vi "EXO2-Sonde Serial thread.vi"() -> ()   [LabVIEW 2016, in "EXO2-Sonde.lvlib"]
uses:
  EXO2-Sonde.lvlib
  <vilib>/Utility/miscctls.llb/LVPointTypeDef.ctl
  Var/Holding Var.vi
  <vilib>/Instr/_visa.llb/VISA Configure Serial Port (Instr).vi
  Var/Input Var.vi
panel:
  in  "停止按钮":bool
  in  "启动按钮":bool
  in  "baud rate (9600)":u32=38400
  out "EXO message":T1
  out "EXO原始数据包":string
  out "收到监测数据":bool
  in  "EXO串口":refnum<visa-resource-name>="COM4"
  in  "EXO启用":bool
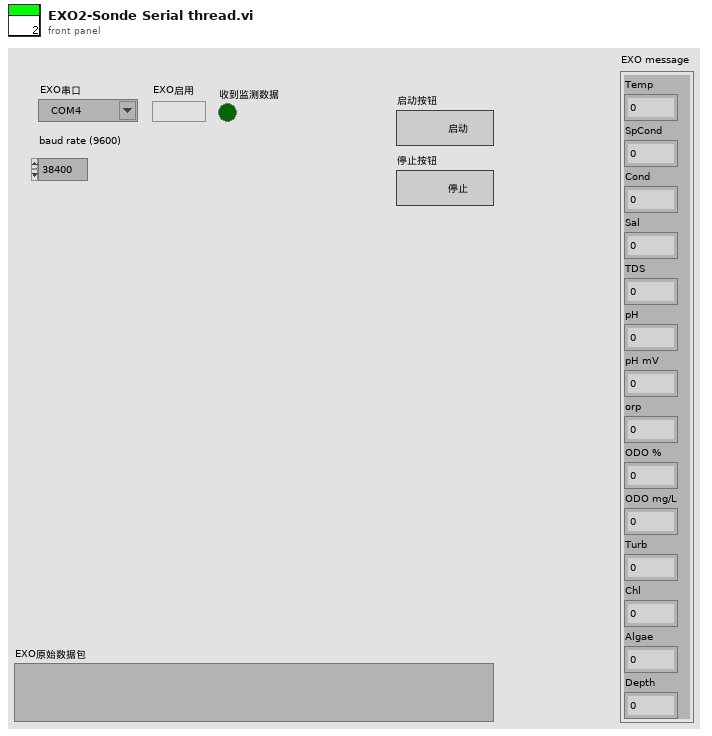
[diagram p1: front panel]
types:
  T1 = cluster{"Temp":dbl, "SpCond":dbl, "Cond":dbl, "Sal":dbl, "TDS":dbl, "pH":dbl, "pH mV":dbl, "orp":dbl, "ODO %":dbl, "ODO mg/L":dbl, "Turb":dbl, "Chl":dbl, "Algae":dbl, "Depth":dbl}
  T2 = enum8{"Enabled", "Disabled", "Disabled and Grayed Out"}
  T3 = typedef "LVPointTypeDef.ctl" = cluster{"Horizontal":i16, "Vertical":i16}
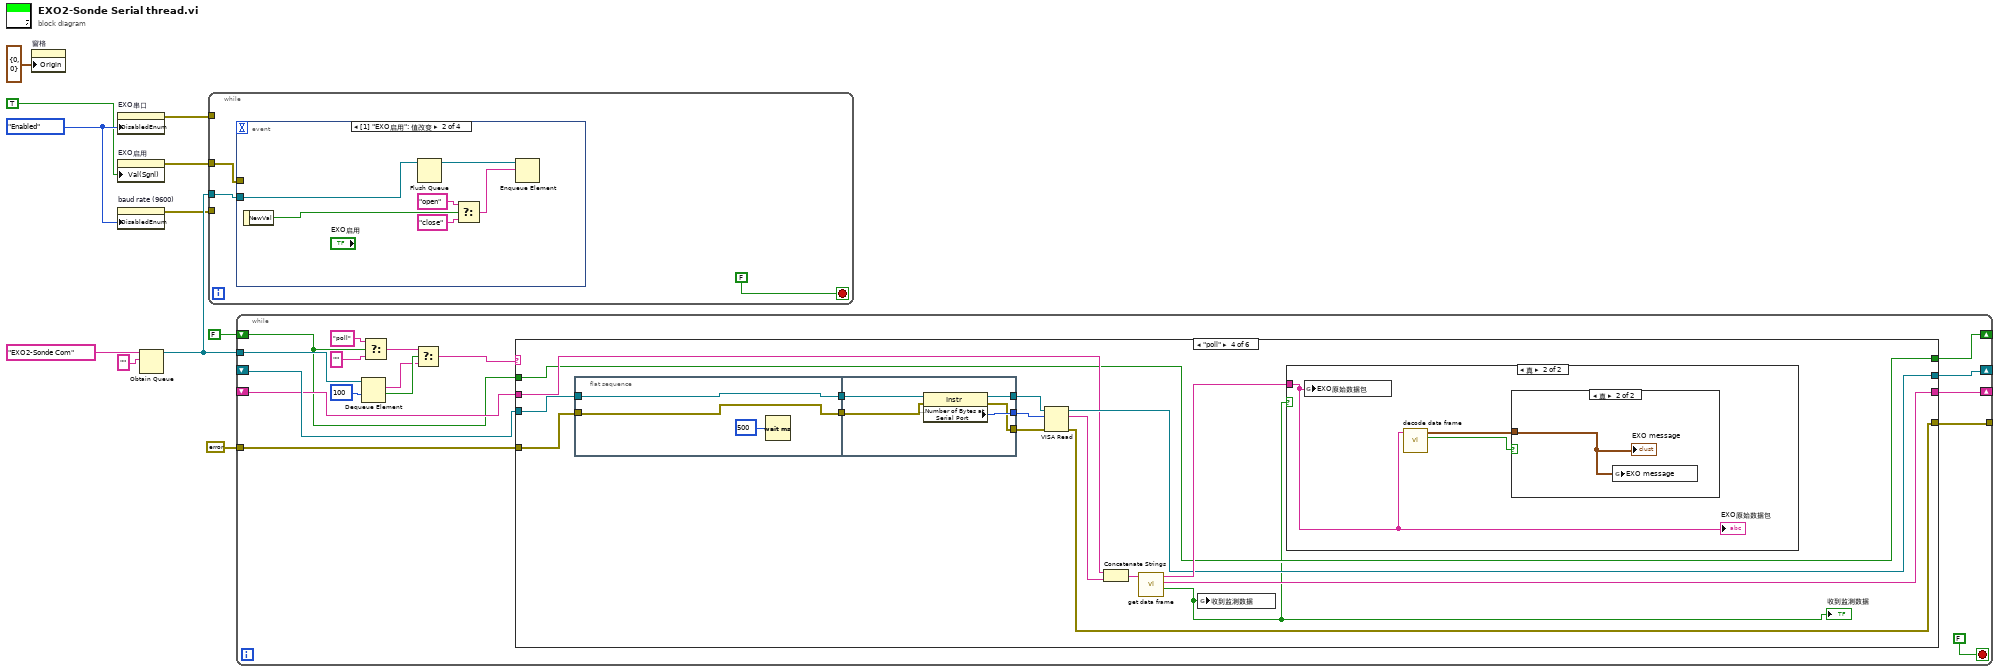
[diagram p0: block diagram]
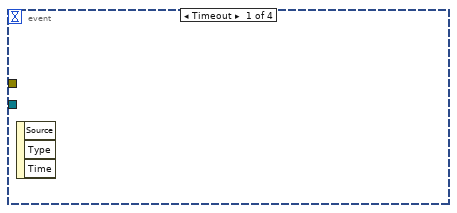
[diagram p2: hidden frame]
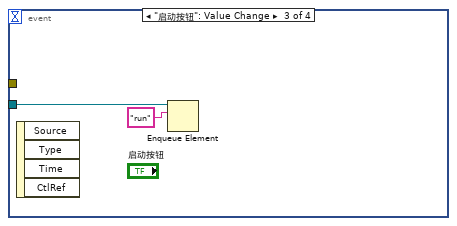
[diagram p3: hidden frame]
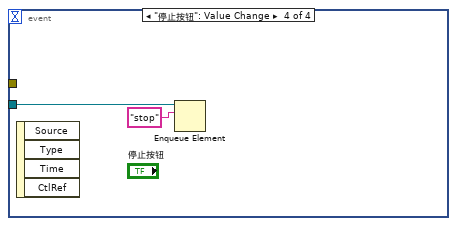
[diagram p4: hidden frame]
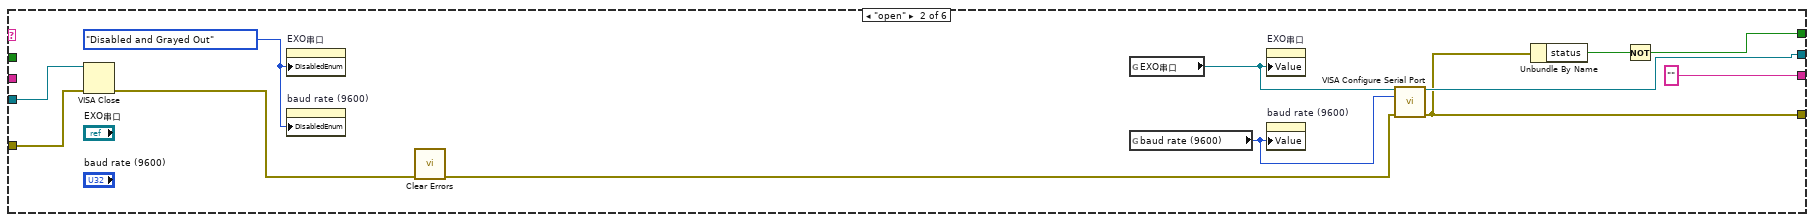
[diagram p6: hidden frame]
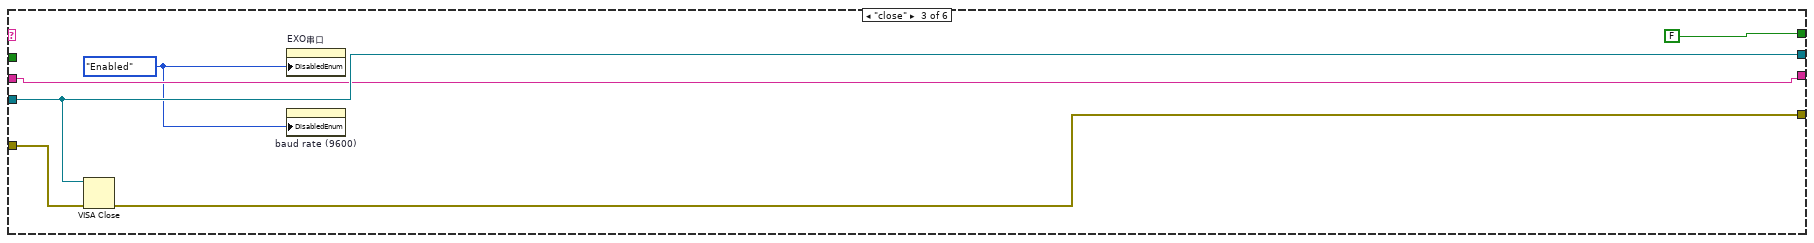
[diagram p7: hidden frame]
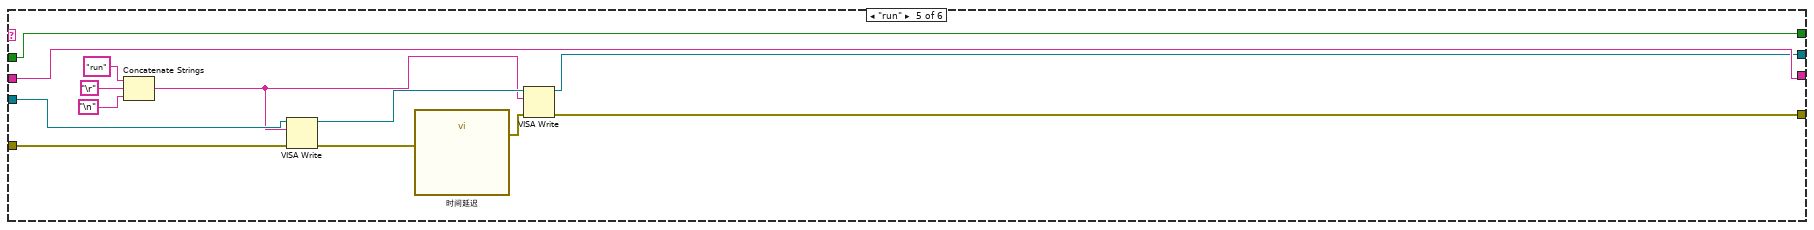
[diagram p10: hidden frame]
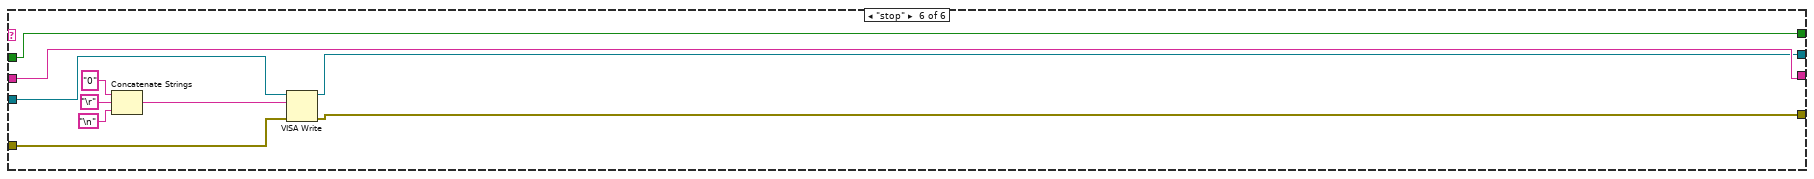
[diagram p11: hidden frame]
diagram:
  w5 = T2."Enabled" ("禁用")
  n1 = property on="窗格" class="Pane"("Origin"=T3 {"Horizontal"=0, "Vertical"=0} ("原点")) -> ()  [unwired: 2 in, 2 out]
  n2 = property on="EXO串口" class="VISAName"("DisabledEnum"=w5) -> (error out=w6:errorcluster)  [unwired: 2 in, 1 out]
  n3 = property on="EXO启用" class="Bool (严格)"("Val(Sgnl)"=TRUE ("值(信号)")) -> (error out=w2:errorcluster)  [unwired: 2 in, 1 out]
  n4 = property on="baud rate (9600)" class="DigNum (严格)"("DisabledEnum"=w5) -> (error out=w4:errorcluster)  [unwired: 2 in, 1 out]
  n5 = Obtain Queue(name (unnamed)="EXO2-Sonde Com" ("名称（未命名）"), element data type="") -> (queue out=w8:refnum<queue>)  [unwired: 3 in, 2 out]
  n6 = while {
    tunnel: w8 -> [w13]
    tunnel: w6 -> [_]
    tunnel: w4 -> [_]
    tunnel: w2 -> [w12]
    stop <- FALSE stop-if-true
    n7 = event shown="[1] \"EXO启用\": 值改变" {
      selector: _ -> [_ _ _ _]
      dyn-events: _ -> [_ _ _ _]
      timeout: _ -> [_ _ _ _]
      tunnel: w13 -> [_ w20 w22 w24]
      tunnel: w12 -> [_ _ _ _]
      event Timeout {
        n8 = event-data() -> ()  [unwired: 1 in, 3 out]
      }
      event "EXO启用": Value Change {
        n9 = event-data() -> ("NewVal"=w19:bool)  [unwired: 1 in]
        n10 = Flush Queue(queue=w20) -> (queue out=w16:refnum<queue>)  [unwired: 1 in, 2 out]
        n11 = Select(t="open", s=w19, f="close") -> (s? t:f=w15:string)
        n12 = Enqueue Element(queue=w16, element=w15) -> ()  [unwired: 2 in, 3 out]
      }
      event "启动按钮": Value Change {
        n13 = event-data() -> ()  [unwired: 1 in, 4 out]
        n14 = Enqueue Element(queue=w22, element="run" ("元素")) -> ()  [unwired: 2 in, 3 out]
      }
      event "停止按钮": Value Change {
        n15 = event-data() -> ()  [unwired: 1 in, 4 out]
        n16 = Enqueue Element(queue=w24, element="stop" ("元素")) -> ()  [unwired: 2 in, 3 out]
      }
    }
  }
  n17 = while {
    tunnel: w8 -> [w40]
    shift-right: [w39] -> _
    shift-left: _ -> [w38]
    shift-right: [w34] -> _
    shift-left: _ -> [w35]
    shift-right: [w33] -> _
    shift-left: FALSE -> [w28]
    tunnel: errorcluster {"status"=FALSE, "code"=0, "source"=""} ("error in (no error)") -> [w36]
    tunnel: [w37] -> _
    stop <- FALSE stop-if-true
    n18 = Dequeue Element(queue=w40, timeout in ms (-1)=100 ("超时毫秒(-1)")) -> (element=w30:string, timed out?=w31:bool)  [unwired: 1 in, 2 out]
    n19 = Select(t="poll", s=w28, f="") -> (s? t:f=w25:string)
    n20 = Select(t=w25, s=w31, f=w30) -> (s? t:f=w29:string)
    n21 = case shown="\"poll\"" w29 {
      tunnel: [w45 w57 w61 w70 w93 w109] -> w39
      tunnel: w38 -> [w45 w56 w61 w73 w104 w114]
      tunnel: [w44 w50 w62 w69 w98 w108] -> w37
      tunnel: w36 -> [w44 w55 w63 w71 w102 w112]
      tunnel: [w43 "" ("匹配+剩余字符串") w60 w68 w103 w113] -> w34
      tunnel: w35 -> [w43 _ w60 w67 w103 w113]
      tunnel: [w42 w48 FALSE w65 w92 w105] -> w33
      tunnel: w28 -> [w42 _ _ w65 w92 w105]
      frame Default {
      }
      frame "open" {
        w51 = T2."Disabled and Grayed Out" ("禁用")
        n22 = VISA Close(VISA resource name=w56, error in (no error)=w55) -> (error out=w54:errorcluster)
        n23 = property on="EXO串口" class="VISAName"("DisabledEnum"=w51) -> ()  [unwired: 2 in, 2 out]
        n24 = property on="baud rate (9600)" class="DigNum (严格)"("DisabledEnum"=w51) -> ()  [unwired: 2 in, 2 out]
        n25 = call <vilib>:"Clear Errors.vi"("error in (no error)"=w54) -> ("error out"=w53:errorcluster)  [unwired: 5 in, 1 out]
        n26 = global read "Holding Var.vi" "EXO串口"() -> (w47:refnum<visa-resource-name>)
        n27 = global read "Holding Var.vi" "baud rate (9600)"() -> (w46:u32)
        n28 = property on="EXO串口" class="VISAName"("Value"=w47) -> ()  [unwired: 2 in, 2 out]
        n29 = property on="baud rate (9600)" class="DigNum (严格)"("Value"=w46) -> ()  [unwired: 2 in, 2 out]
        n30 = call-poly "VISA Configure Serial Port"("VISA resource name"=w47, "baud rate (9600)"=w46, "error in (no error)"=w53) -> ("VISA resource name out"=w57:refnum<visa-resource-name>, "error out"=w50:errorcluster)  [unwired: 11 in]
        n31 = Unbundle By Name(w50) -> ("status"=w49:bool)
        n32 = Not(x=w49) -> (.not. x?=w48:bool)
      }
      frame "close" {
        w59 = T2."Enabled" ("禁用")
        n33 = VISA Close(VISA resource name=w61, error in (no error)=w63) -> (error out=w62:errorcluster)
        n34 = property on="EXO串口" class="VISAName"("DisabledEnum"=w59) -> ()  [unwired: 2 in, 2 out]
        n35 = property on="baud rate (9600)" class="DigNum (严格)"("DisabledEnum"=w59) -> ()  [unwired: 2 in, 2 out]
      }
      frame "poll" {
        n36 = flat-sequence {
          tunnel: [w85] -> w74
          tunnel: w73 -> [w85]
          tunnel: [w84] -> w72
          tunnel: w71 -> [w84]
          tunnel: [w91] -> w75
          tunnel: [w90] -> w76
          tunnel: [w89] -> w77
          tunnel: w74 -> [w88]
          tunnel: w72 -> [w87]
          frame #0 {
            n37 = Wait (ms)(milliseconds to wait=u32 500 ("等待时间（毫秒）")) -> ()  [unwired: 1 out]
          }
          frame #1 {
            n38 = property class="Instr"(reference=w88, error in=w87) -> (reference out=w91:refnum<visa-resource-name>, error out=w89:errorcluster, "Serial Settings:Number of Bytes at Serial Port"=w90:u32)
          }
        }
        n39 = VISA Read(VISA resource name=w75, byte count=w76, error in (no error)=w77) -> (VISA resource name out=w70:refnum<visa-resource-name>, read buffer=w78:string, error out=w69:errorcluster)  [unwired: 1 out]
        n40 = Concatenate Strings(w67, w78) -> (w66:string)
        n41 = call "get data frame.vi"("字符串"=w66) -> ("标记位"=w64:bool, "匹配+剩余字符串"=w68:string, "匹配之前的子字符串"=w79:string)  [unwired: 8 in]
        "收到监测数据" <- w64
        n42 = global write "Input Var.vi" "收到监测数据"(w64) -> ()
        n43 = case shown="真" w64 {
          tunnel: w79 -> [_ w81]
          frame False {
          }
          frame True {
            n44 = global write "Input Var.vi" "EXO原始数据包"(w81) -> ()
            n45 = call "decode data frame.vi"("字符串"=w81) -> ("x >= y?"=w80:bool, "EXO message"=w82:T1)  [unwired: 9 in]
            n46 = case shown="真" w80 {
              tunnel: w82 -> [_ w83]
              frame False {
              }
              frame True {
                n47 = global write "Input Var.vi" "EXO message"(w83) -> ()
                "EXO message" <- w83
              }
            }
            "EXO原始数据包" <- w81
          }
        }
      }
      frame "run" {
        n48 = Concatenate Strings("run" ("写入缓冲区"), "\r", "\n") -> (w94:string)
        n49 = VISA Write(VISA resource name=w104, write buffer=w94, error in (no error)=w102) -> (VISA resource name out=w95:refnum<visa-resource-name>, error out=w97:errorcluster)  [unwired: 1 out]
        n50 = call "时间延迟"("error in (no error)"=w97) -> ("error out"=w96:errorcluster)  [unwired: 10 in]
        n51 = VISA Write(VISA resource name=w95, write buffer=w94, error in (no error)=w96) -> (VISA resource name out=w93:refnum<visa-resource-name>, error out=w98:errorcluster)  [unwired: 1 out]
      }
      frame "stop" {
        n52 = Concatenate Strings("0" ("写入缓冲区"), "\r", "\n") -> (w110:string)
        n53 = VISA Write(VISA resource name=w114, write buffer=w110, error in (no error)=w112) -> (VISA resource name out=w109:refnum<visa-resource-name>, error out=w108:errorcluster)  [unwired: 1 out]
      }
    }
  }
